vi "RT Driver VI.vi"(6 "Device Clock":string, 9 "Device Inputs FIFO":refnum<k33>, 10 "Device Outputs FIFO":refnum<k33>, 11 "Device Reference":T1 format="%.0x") -> ()   [LabVIEW 2021, in "G5 Regatron Custom Device Engine.lvlib"]
uses:
  G5 Regatron Custom Device Engine.lvlib
  <vilib>/NI VeriStand/Custom Device API/Custom Device Item Ref.ctl
  <vilib>/NI VeriStand/Custom Device API/Custom Device Channel Type.ctl
  <vilib>/Platform/TimedLoop/XDataNode/nitl_modes.ctl
  Shared/Regatron.G5.Rest Handle.llb/G5.Rest Status.ctl
  Shared/Regatron.G5.Rest System.llb/G5.Rest System Output References Datasource.ctl
  Shared/Regatron.G5.Rest System.llb/G5.Rest System Output Limits Datasource.ctl
  Shared/Regatron.G5.Rest Config.llb/G5.Rest Config Sensing Observation Datasource.ctl
  Shared/G5.Rest Battery Control Functions.ctl
  Shared/Regatron.G5.Rest System.llb/G5.Rest System Output Limits.ctl
  Shared/Regatron.G5.Rest System.llb/G5.Rest System Output References.ctl
  Shared/Regatron.G5.Rest System.llb/G5.Rest System Clear Inicidents.ctl
  Shared/Regatron.G5.Rest Config.llb/G5.Rest Sensing Observation References.ctl
  Shared/G5.Rest Battery Control Values.ctl
  <userlib>/_OpenG.lib/array/array.llb/Search 1D Array (Boolean)__ogtk.vi
  <vilib>/NI VeriStand/Custom Device API/Custom Device API.lvlib
  <vilib>/NI VeriStand/Custom Device Tools/Custom Device Utility Library/Custom Device Utility Library.lvlib
  <vilib>/Platform/TimedLoop/XDataNode/XDNodeRunTimeDep.lvlib
  Shared/Regatron.G5.Rest.lvlib
panel:
  in  "Initialization Status Notifier":refnum<notifier>
  in  "Status Notifier":refnum<notifier>
  # "Custom Device Template\nv1.0"
  # "Use this template as a starting point for creating a custom device code module. The input controls shown here are specially named controls that the system will use to provide the device loop with data. The controls are not required for the device loop to run. For instance, if the device doesn't produce any output data, then you don't need the Device Outputs FIFO control. If you do use these controls, however, they need to have these exact names to be functional."
  # "The optional status notifier element is used to notify the RT engine of the last state of the custom device, and to indicate the device has completed execution. If this control is not used, a default No Error value is returned to the system when the device finishes execution.\n\nNote: This error state is not checked until the system shuts down. Use an output status channel to send more immediate status values to the system."
  # "This optional input can be used to send the VeriStand Engine the final status of the custom device initalization process. If this control exists on the custom device front panel, the VeriStand Engine will wait for a status update before starting up. If the custom device reports an error, that will abort the execution of the current configuration in the VeriStand Engine.\n\nThis control can be deleted if the custom device does not need to send the initialization status update."
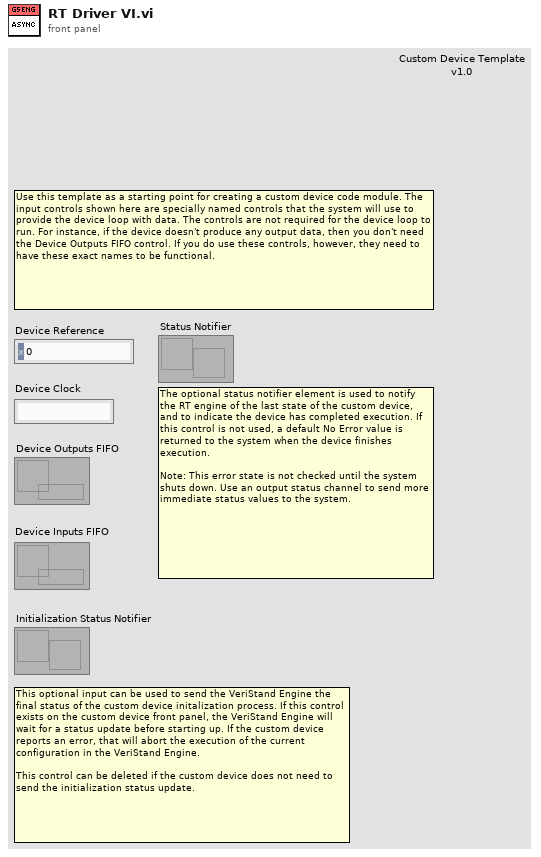
[diagram p1: front panel]
types:
  T1 = typedef "Custom Device API.lvlib/Custom Device Item Ref.ctl" = u64
  T2 = typedef "Custom Device API.lvlib/Custom Device Channel Type.ctl" = enum16{"Input", "Output"}
  T3 = typedef "Custom Device API.lvlib/Custom Device Timed Loop Priority.ctl" = enum32{"Low", "Medium", "High"}
  T4 = typedef "Regatron.G5.Rest.lvlib/G5.Rest Status.ctl" = enum16{"Read", "Write"}
  T5 = typedef "Regatron.G5.Rest.lvlib/G5.Rest Battery Control Functions.ctl" = enum16{"Read Energy Count", "Read Charge Count", "Reset Energy Charge Counters"}
  T6 = typedef "Regatron.G5.Rest.lvlib/G5.Rest System Output Limits.ctl" = cluster{"Voltage Upper Limit V":sgl, "Voltage Lower Limit V":sgl, "Current Upper Limit A":sgl, "Current Lower Limit A":sgl, "Power Upper Limit W":sgl, "Power Lower Limit W":sgl}
  T7 = typedef "Regatron.G5.Rest.lvlib/G5.Rest System Output References.ctl" = cluster{"Voltage V":sgl, "Current A":sgl, "Power W":sgl, "Load R Ohm":sgl}
  T8 = typedef "Regatron.G5.Rest.lvlib/G5.Rest System Clear Inicidents.ctl" = enum16{"Clear Errors and Warnings", "Clear Warnings", "Clear Errors"}
  T9 = typedef "Regatron.G5.Rest.lvlib/G5.Rest Sensing Observation References.ctl" = cluster{"Voltage Max Level (V)":sgl, "Voltage Max Delay (ms)":sgl}
  T10 = typedef "Regatron.G5.Rest.lvlib/G5.Rest Battery Control Values.ctl" = cluster{"Charge Counter":dbl, "Energy Counter":dbl, "ResetEnergyChargeCounters":dbl}
  T11 = typedef "XDNodeRunTimeDep.lvlib/nitl_modes.ctl" = enum32{"No Change", "Process missed periods, maintain original phase", "Discard missed periods, maintain original phase", "Process missed periods, ignore original phase", "Discard missed periods, ignore original phase"}
  T12 = typedef "Regatron.G5.Rest.lvlib/G5.Rest System Output References Datasource.ctl" = enum16{"Voltage", "Current", "Power", "Load Resistance", "ALL"}[]
  T13 = enum16{"Undefined", "PowerUp", "NotReady", "Ready", "VoltageOnPrepare", "VoltageOn", "VoltageOnLeave", "Test", "FirmwareUpdate"}
  T14 = typedef "Regatron.G5.Rest.lvlib/G5.Rest Config Quadrantmode.ctl" = enum16{"Bidirectional", "Q1 Only", "Q4 Only"}
  T15 = enum16{"VoltageControlled", "CurrentControlled", "PowerControlled", "ResistanceControlled"}
  T16 = typedef "Regatron.G5.Rest.lvlib/G5.Rest System Output Limits Datasource.ctl" = enum16{"Voltage Upper Limit", "Voltage Lower Limit", "Current Upper Limit", "Current Lower Limit", "Power Upper Limit", "Power Lower Limit", "ALL"}[]
  T17 = typedef "Regatron.G5.Rest.lvlib/G5.Rest Config Sensing Observation Datasource.ctl" = enum16{"Voltage Max Level", "Voltage Max Delay", "ALL"}[]
  T18 = typedef "Regatron.G5.Rest.lvlib/G5.Rest System Output Values.ctl" = cluster{"Voltage V":sgl, "Current A":sgl, "Power W":sgl, "Power kW":sgl, "Load R Ohm":sgl}
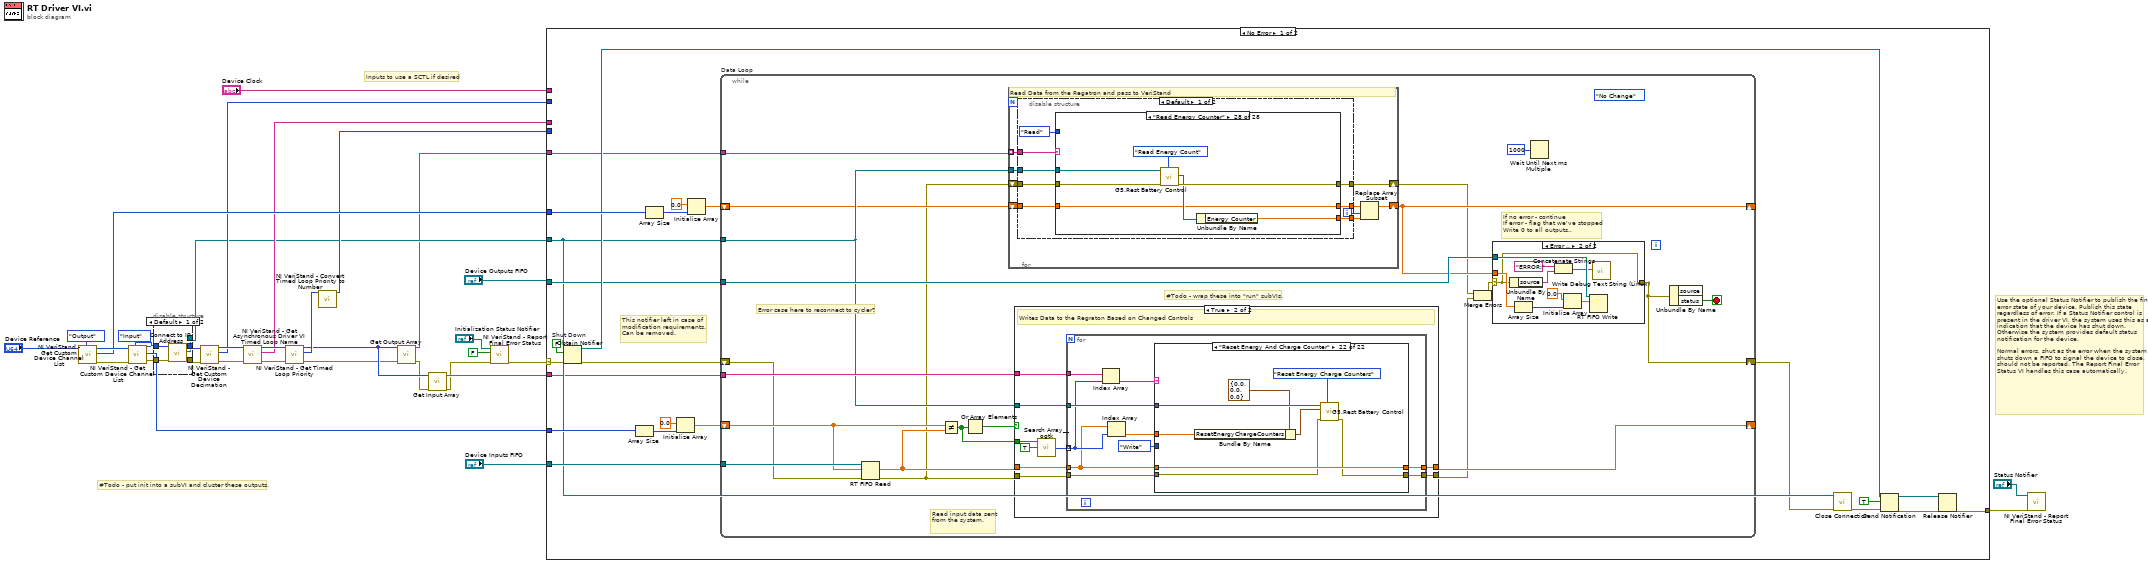
[diagram p0: block diagram]
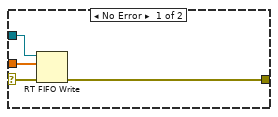
[diagram p3: hidden frame]
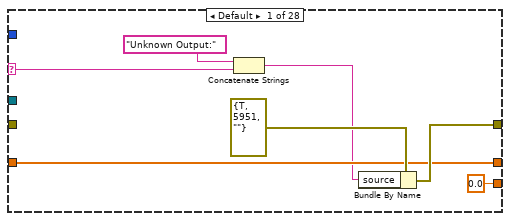
[diagram p4: hidden frame]
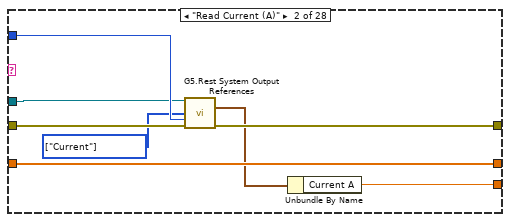
[diagram p5: hidden frame]
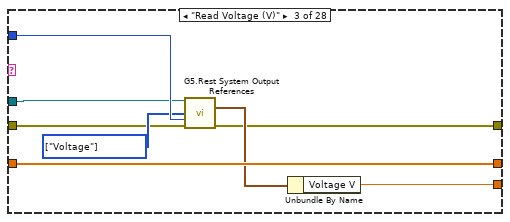
[diagram p6: hidden frame]
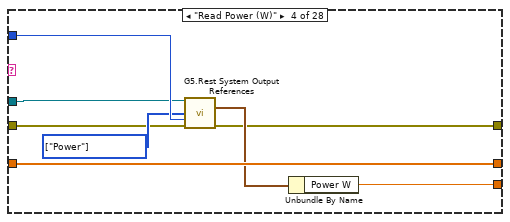
[diagram p7: hidden frame]
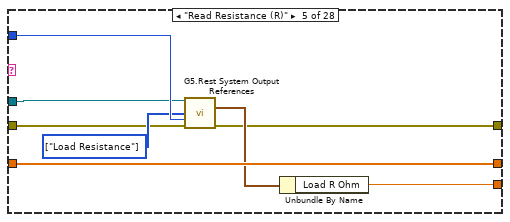
[diagram p8: hidden frame]
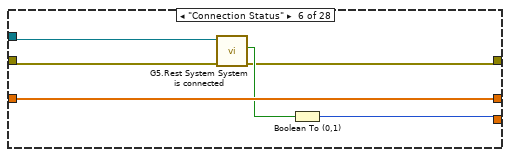
[diagram p9: hidden frame]
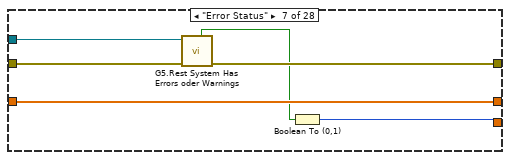
[diagram p10: hidden frame]
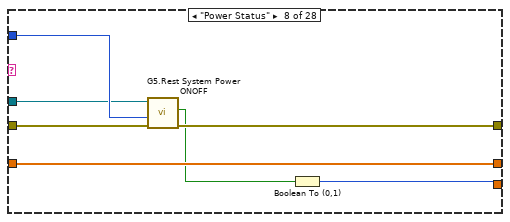
[diagram p11: hidden frame]
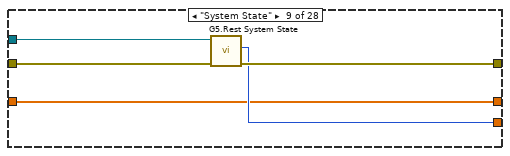
[diagram p12: hidden frame]
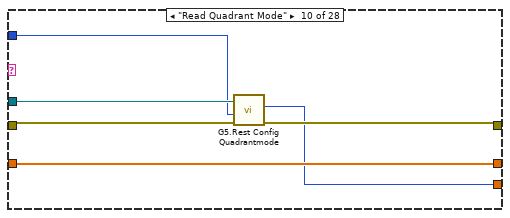
[diagram p13: hidden frame]
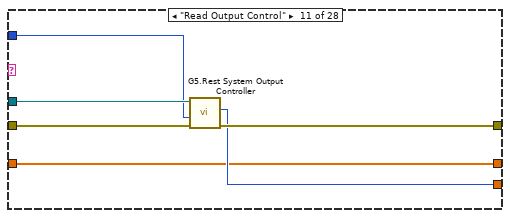
[diagram p14: hidden frame]
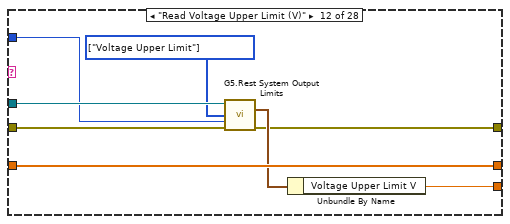
[diagram p15: hidden frame]
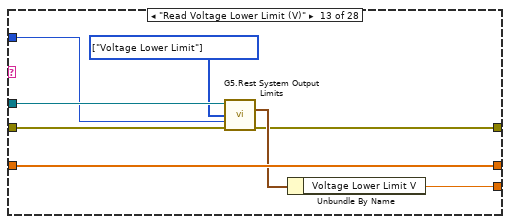
[diagram p16: hidden frame]
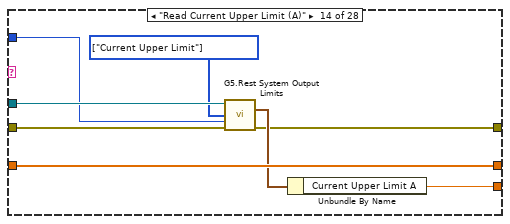
[diagram p17: hidden frame]
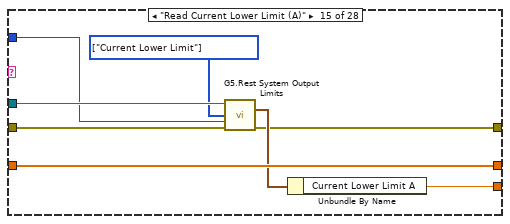
[diagram p18: hidden frame]
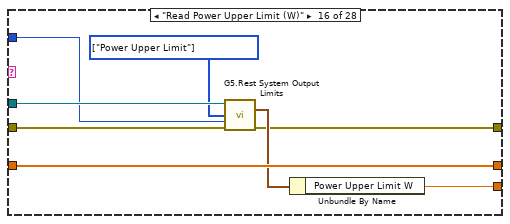
[diagram p19: hidden frame]
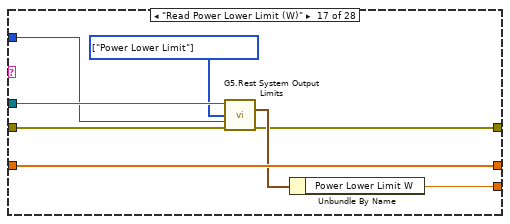
[diagram p20: hidden frame]
diagram:
  # "#Todo - put init into a subVI and cluster these outputs."
  # "Inputs to use a SCTL if desired"
  # "Use the optional Status Notifier to publish the final error state of your device. Publish this state regardless of error. If a Status Notifier control is present in the driver VI, the system uses this as an indication that the device has shut down. Otherwise the system provides default status notification for the device.\n\nNormal errors, shut as the error when the system shuts down a FIFO to signal the device to close, should not be reported. The Report Final Error Status VI handles this case automatically."
  n1 = call <vilib>:"NI VeriStand - Get Custom Device Channel List.vi"("Channel Type"=Custom_Device_Channel_Type."Output", "Device Ref in"="Device Reference") -> ("error out"=w29:errorcluster, "Specified Channel Ref List"=w26:T1[], "Device Ref out"=w30:T1)  [unwired: 1 in, 6 out]
  n2 = call <vilib>:"NI VeriStand - Get Custom Device Channel List.vi"("Channel Type"=Custom_Device_Channel_Type."Input", "error in (no error)"=w29, "Device Ref in"=w30) -> ("error out"=w22:errorcluster, "Specified Channel Ref List"=w27:T1[], "Device Ref out"=w15:T1)  [unwired: 6 out]
  n3 = disable-structure shown="Default" {
    disable-tunnel: w22 -> [w39 w40]
    disable-tunnel: [w38 w40] -> w16
    disable-tunnel: w15 -> [w37 w41]
    disable-tunnel: [w36 w41] -> w14
    disable-tunnel: [w35 _] -> w4
    frame condition #0 (active) {
      n4 = call "Connect to IP Address.vi"("error in (no error)"=w39, "Device Ref in"=w37) -> ("error out"=w38:errorcluster, "REST Client out"=w35:refnum<class "REST Client.lvclass">, "Item Ref out"=w36:T1)  [unwired: 7 in]
    }
    frame condition #1 {
    }
  }
  n5 = call <vilib>:"NI VeriStand - Get Custom Device Decimation.vi"("error in (no error)"=w16, "Device Ref in"=w14) -> ("error out"=w20:errorcluster, "Decimation"=w12:i32, "Device Ref out"=w21:T1)  [unwired: 7 in]
  n6 = call <vilib>:"NI VeriStand - Get Asynchronous Driver VI Timed Loop Name.vi"("error in (no error)"=w20, "Device Ref in"=w21) -> ("error out"=w19:errorcluster, "Device Timed Loop Name"=w11:string, "Device Ref out"=w18:T1)  [unwired: 7 in]
  n7 = call <vilib>:"NI VeriStand - Get Timed Loop Priority.vi"("error in (no error)"=w19, "Device Ref in"=w18) -> ("error out"=w8:errorcluster, "Priority"=w17:T3, "Device Ref out"=w9:T1)  [unwired: 7 in]
  n8 = call <vilib>:"NI VeriStand - Convert Timed Loop Priority to Number.vi"("Priority"=w17) -> ("Numeric Priority"=w10:i32)  [unwired: 10 in]
  n9 = call "Get Output Array.vi"("error in"=w8, "Device Ref in"=w9) -> ("error out"=w7:errorcluster, "Array"=w1:string[])  [unwired: 8 in]
  n10 = call "Get Input Array.vi"("error in"=w7, "Device Ref in"=w9) -> ("error out"=w5:errorcluster, "Array"=w6:string[])  [unwired: 8 in]
  n11 = call <vilib>:"NI VeriStand - Report Final Error Status.vi"("error in (no error)"=w5, "Filter FIFO & Shutdown Errors (T)"=FALSE ("Filter FIFO Errors (T)"), "Status Notifier"="Initialization Status Notifier") -> ("error out"=w3:errorcluster)  [unwired: 8 out]
  n12 = case shown="No Error" w3 {
    selector: w3 -> [w56 w512]
    tunnel: "Device Outputs FIFO" -> [w50 _]
    tunnel: "Device Inputs FIFO" -> [w52 _]
    tunnel: w27 -> [w61 _]
    tunnel: w26 -> [w60 _]
    tunnel: [w43 w512] -> w2
    tunnel: "Device Clock" -> [_ _]
    tunnel: w12 -> [_ _]
    tunnel: w11 -> [_ _]
    tunnel: w10 -> [_ _]
    tunnel: w1 -> [w42 _]
    tunnel: w6 -> [w44 _]
    tunnel: w4 -> [w46 _]
    frame No Error {
      w58 = FALSE  # Shut Down
      # "This notifier left in case of \nmodification requirements.\nCan be removed."
      n13 = Obtain Notifier(notification data type=w58, error in (no error)=w56) -> (notifier out=w57:refnum<notifier>, error out=w49:errorcluster)  [unwired: 2 in, 1 out]
      n14 = Array Size(array=w61) -> (size(s)=w59:i32)
      n15 = Array Size(array=w60) -> (size(s)=w62:i32)
      n16 = Initialize Array(0.0 ("element"), w59) -> (w53:dbl[])
      n17 = Initialize Array(0.0 ("element"), w62) -> (w51:dbl[])
      n18 = while "Data Loop" {
        shift-right: [w84] -> _
        shift-left: w53 -> [w81]
        shift-right: [w70] -> w45
        shift-left: w49 -> [w69]
        shift-right: [w73] -> _
        shift-left: w51 -> [w74]
        tunnel: w50 -> [w83]
        tunnel: w52 -> [w82]
        tunnel: w46 -> [w75]
        tunnel: w44 -> [w80]
        tunnel: w42 -> [w76]
        stop <- w72 stop-if-true
        (unwired) nitl_modes."No Change" ("Mode")
        # "Error case here to reconnect to cycler?"
        # "If no error - continue\nIf error - flag that we've stopped\nWrite 0 to all outputs.."
        # "#Todo - wrap these into \"run\" subVIs."
        # "Read input data sent from the system."
        n19 = RT FIFO Read(0:w82, 1:w81, 3:w69) -> (9:w78:dbl[], 11:w68:errorcluster)  [unwired: 4 out]
        n20 = Not Equal?(x=w81, y=w78) -> (x != y?=w79:bool[])
        n21 = Or Array Elements(Boolean array=w79) -> (logical OR=w77:bool)
        n22 = for {
          tunnel: w76 -> [w98] mode=indexing
          tunnel: w75 -> [w106]
          shift-right: [w105] -> w66
          shift-left: w68 -> [w103]
          shift-right: [w99] -> w73
          shift-left: w74 -> [w104]
          i -> [w101]
          # "Read Data from the Regatron and pass to VeriStand"
          n23 = disable-structure shown="Default" {
            disable-tunnel: w106 -> [w114 _]
            disable-tunnel: [w113 w315] -> w105
            disable-tunnel: w104 -> [w112 w316]
            disable-tunnel: w103 -> [w111 w315]
            disable-tunnel: [w110 w316] -> w102
            disable-tunnel: [w109 _] -> w100
            disable-tunnel: w98 -> [w107 w317]
            frame condition #0 (active) {
              n24 = case shown="\"Read Energy Counter\"" w107 {
                selector: w107 -> [w116 _ _ _ _ _ _ _ _ _ _ _ _ _ _ _ _ _ _ _ _ _ _ _ _ _ _ _]
                tunnel: w114 -> [_ w125 w131 w139 w147 w157 w163 w169 w177 w183 w189 w197 w205 w213 w221 w229 w237 w244 w249 w256 w264 w272 w279 w286 w293 w300 w307 w314]
                tunnel: w111 -> [_ w126 w132 w140 w148 w156 w162 w168 w176 w181 w188 w196 w204 w212 w220 w228 w236 w243 w248 w255 w263 w271 w278 w285 w292 w299 w305 w312]
                tunnel: [w120 w124 w130 w138 w146 w154 w161 w167 w175 w180 w186 w190 w198 w206 w214 w222 w230 w241 w247 w254 w260 w268 w277 w282 w289 w296 w304 w311] -> w113
                tunnel: w112 -> [w118 w129 w137 w145 w153 w159 w165 w172 w173 w179 w184 w193 w201 w209 w217 w225 w233 w238 w245 w251 w258 w266 w275 w280 w287 w294 w302 w309]
                tunnel: [w118 w129 w137 w145 w153 w159 w165 w172 w173 w179 w184 w193 w201 w209 w217 w225 w233 w238 w245 w251 w258 w266 w275 w280 w287 w294 w302 w309] -> w110
                tunnel: [sgl 0.0 ("Load R Ohm") w128 w135 w143 w151 w158 w164 w171 w174 w178 w185 w191 w199 w207 w215 w223 w231 w239 w246 w252 w257 w265 w276 w281 w288 w295 w301 w308] -> w109
                tunnel: G5.Rest_Status."Read" ("Status") -> [_ w127 w134 w142 w150 _ _ w170 _ w182 w187 w195 w203 w211 w219 w227 w235 w242 w250 _ w262 w270 _ _ _ _ _ _]
                frame Default {
                  n25 = Concatenate Strings("Unknown Output:" ("string"), w116) -> (w115:string)
                  n26 = Bundle By Name(cluster=errorcluster {"status"=TRUE, "code"=5951, "source"=""} ("Fehler (Ausgang)"), "source"=w115) -> (w120:errorcluster)
                }
                frame "Read Current (A)" {
                  w122 = T12 [enum."Current"] items=["Voltage", "Current", "Power", "Load Resistance", "ALL"] ("Datasource")
                  n27 = call "G5.Rest System Output References .vi"("G5 WEB API (Eingang)"=w125, "Datasource"=w122, "Status"=w127, "Fehler (Eingang, kein Fehler)"=w126) -> ("GET Output Reference"=w123:T7, "Fehler (Ausgang)"=w124:errorcluster)  [unwired: 9 in, 1 out]
                  n28 = Unbundle By Name(w123) -> ("Current A"=w128:sgl)
                }
                frame "Read Voltage (V)" {
                  w133 = T12 [enum."Voltage"] items=["Voltage", "Current", "Power", "Load Resistance", "ALL"] ("Datasource")
                  n29 = call "G5.Rest System Output References .vi"("G5 WEB API (Eingang)"=w131, "Datasource"=w133, "Status"=w134, "Fehler (Eingang, kein Fehler)"=w132) -> ("GET Output Reference"=w136:T7, "Fehler (Ausgang)"=w130:errorcluster)  [unwired: 9 in, 1 out]
                  n30 = Unbundle By Name(w136) -> ("Voltage V"=w135:sgl)
                }
                frame "Read Power (W)" {
                  w141 = T12 [enum."Power"] items=["Voltage", "Current", "Power", "Load Resistance", "ALL"] ("Datasource")
                  n31 = call "G5.Rest System Output References .vi"("G5 WEB API (Eingang)"=w139, "Datasource"=w141, "Status"=w142, "Fehler (Eingang, kein Fehler)"=w140) -> ("GET Output Reference"=w144:T7, "Fehler (Ausgang)"=w138:errorcluster)  [unwired: 9 in, 1 out]
                  n32 = Unbundle By Name(w144) -> ("Power W"=w143:sgl)
                }
                frame "Read Resistance (R)" {
                  w149 = T12 [enum."Load Resistance"] items=["Voltage", "Current", "Power", "Load Resistance", "ALL"] ("Datasource")
                  n33 = call "G5.Rest System Output References .vi"("G5 WEB API (Eingang)"=w147, "Datasource"=w149, "Status"=w150, "Fehler (Eingang, kein Fehler)"=w148) -> ("GET Output Reference"=w152:T7, "Fehler (Ausgang)"=w146:errorcluster)  [unwired: 9 in, 1 out]
                  n34 = Unbundle By Name(w152) -> ("Load R Ohm"=w151:sgl)
                }
                frame "Connection Status" {
                  n35 = call "G5.Rest System System is connected.vi"("Fehler (Eingang, kein Fehler)"=w156, "G5 WEB API (Eingang)"=w157) -> ("Fehler (Ausgang)"=w154:errorcluster, "System is connected"=w155:bool)  [unwired: 7 in, 1 out]
                  n36 = Boolean To (0,1)(Boolean=w155) -> (0, 1=w158:i16)
                }
                frame "Error Status" {
                  n37 = call "G5.Rest System Has Errors oder Warnings.vi"("Fehler (Eingang, kein Fehler)"=w162, "G5 WEB API (Eingang)"=w163) -> ("Fehler (Ausgang)"=w161:errorcluster, "System has Errors or Warnings"=w160:bool)  [unwired: 5 in, 3 out]
                  n38 = Boolean To (0,1)(Boolean=w160) -> (0, 1=w164:i16)
                }
                frame "Power Status" {
                  n39 = call "G5.Rest System Power ONOFF.vi"("Fehler (Eingang, kein Fehler)"=w168, "Status"=w170, "G5 WEB API (Eingang)"=w169) -> ("Fehler (Ausgang)"=w167:errorcluster, "Get Power OFF/ON"=w166:bool)  [unwired: 6 in, 1 out]
                  n40 = Boolean To (0,1)(Boolean=w166) -> (0, 1=w171:i16)
                }
                frame "System State" {
                  n41 = call "G5.Rest System State.vi"("Fehler (Eingang, kein Fehler)"=w176, "G5 WEB API (Eingang)"=w177) -> ("Fehler (Ausgang)"=w175:errorcluster, "GET State"=w174:T13)  [unwired: 7 in, 1 out]
                }
                frame "Read Quadrant Mode" {
                  n42 = call "G5.Rest Config Quadrantmode.vi"("Fehler (Eingang, kein Fehler)"=w181, "Status"=w182, "G5 WEB API (Eingang)"=w183) -> ("Fehler (Ausgang)"=w180:errorcluster, "GET Quadrant Mode"=w178:T14)  [unwired: 6 in, 1 out]
                }
                frame "Read Output Control" {
                  n43 = call "G5.Rest System Output Controller.vi"("Fehler (Eingang, kein Fehler)"=w188, "Status"=w187, "G5 WEB API (Eingang)"=w189) -> ("Fehler (Ausgang)"=w186:errorcluster, "GET Output Control"=w185:T15)  [unwired: 6 in, 1 out]
                }
                frame "Read Voltage Upper Limit (V)" {
                  w194 = T16 [enum."Voltage Upper Limit"] items=["Voltage Upper Limit", "Voltage Lower Limit", "Current Upper Limit", "Current Lower Limit", "Power Upper Limit", "Power Lower Limit", "ALL"] ("Datasource")
                  n44 = call "G5.Rest System Output Limits.vi"("G5 WEB API (Eingang)"=w197, "Datasource"=w194, "Status"=w195, "Fehler (Eingang, kein Fehler)"=w196) -> ("GET Output Limit"=w192:T6, "Fehler (Ausgang)"=w190:errorcluster)  [unwired: 9 in, 1 out]
                  n45 = Unbundle By Name(w192) -> ("Voltage Upper Limit V"=w191:sgl)
                }
                frame "Read Voltage Lower Limit (V)" {
                  w202 = T16 [enum."Voltage Lower Limit"] items=["Voltage Upper Limit", "Voltage Lower Limit", "Current Upper Limit", "Current Lower Limit", "Power Upper Limit", "Power Lower Limit", "ALL"] ("Datasource")
                  n46 = call "G5.Rest System Output Limits.vi"("G5 WEB API (Eingang)"=w205, "Datasource"=w202, "Status"=w203, "Fehler (Eingang, kein Fehler)"=w204) -> ("GET Output Limit"=w200:T6, "Fehler (Ausgang)"=w198:errorcluster)  [unwired: 9 in, 1 out]
                  n47 = Unbundle By Name(w200) -> ("Voltage Lower Limit V"=w199:sgl)
                }
                frame "Read Current Upper Limit (A)" {
                  w210 = T16 [enum."Current Upper Limit"] items=["Voltage Upper Limit", "Voltage Lower Limit", "Current Upper Limit", "Current Lower Limit", "Power Upper Limit", "Power Lower Limit", "ALL"] ("Datasource")
                  n48 = call "G5.Rest System Output Limits.vi"("G5 WEB API (Eingang)"=w213, "Datasource"=w210, "Status"=w211, "Fehler (Eingang, kein Fehler)"=w212) -> ("GET Output Limit"=w208:T6, "Fehler (Ausgang)"=w206:errorcluster)  [unwired: 9 in, 1 out]
                  n49 = Unbundle By Name(w208) -> ("Current Upper Limit A"=w207:sgl)
                }
                frame "Read Current Lower Limit (A)" {
                  w218 = T16 [enum."Current Lower Limit"] items=["Voltage Upper Limit", "Voltage Lower Limit", "Current Upper Limit", "Current Lower Limit", "Power Upper Limit", "Power Lower Limit", "ALL"] ("Datasource")
                  n50 = call "G5.Rest System Output Limits.vi"("G5 WEB API (Eingang)"=w221, "Datasource"=w218, "Status"=w219, "Fehler (Eingang, kein Fehler)"=w220) -> ("GET Output Limit"=w216:T6, "Fehler (Ausgang)"=w214:errorcluster)  [unwired: 9 in, 1 out]
                  n51 = Unbundle By Name(w216) -> ("Current Lower Limit A"=w215:sgl)
                }
                frame "Read Power Upper Limit (W)" {
                  w226 = T16 [enum."Power Upper Limit"] items=["Voltage Upper Limit", "Voltage Lower Limit", "Current Upper Limit", "Current Lower Limit", "Power Upper Limit", "Power Lower Limit", "ALL"] ("Datasource")
                  n52 = call "G5.Rest System Output Limits.vi"("G5 WEB API (Eingang)"=w229, "Datasource"=w226, "Status"=w227, "Fehler (Eingang, kein Fehler)"=w228) -> ("GET Output Limit"=w224:T6, "Fehler (Ausgang)"=w222:errorcluster)  [unwired: 9 in, 1 out]
                  n53 = Unbundle By Name(w224) -> ("Power Upper Limit W"=w223:sgl)
                }
                frame "Read Power Lower Limit (W)" {
                  w234 = T16 [enum."Power Lower Limit"] items=["Voltage Upper Limit", "Voltage Lower Limit", "Current Upper Limit", "Current Lower Limit", "Power Upper Limit", "Power Lower Limit", "ALL"] ("Datasource")
                  n54 = call "G5.Rest System Output Limits.vi"("G5 WEB API (Eingang)"=w237, "Datasource"=w234, "Status"=w235, "Fehler (Eingang, kein Fehler)"=w236) -> ("GET Output Limit"=w232:T6, "Fehler (Ausgang)"=w230:errorcluster)  [unwired: 9 in, 1 out]
                  n55 = Unbundle By Name(w232) -> ("Power Lower Limit W"=w231:sgl)
                }
                frame "Read Sense Enable" {
                  n56 = call "G5.Rest Config Sensing Enable.vi"("Fehler (Eingang, kein Fehler)"=w243, "Status"=w242, "G5 WEB API (Eingang)"=w244) -> ("Fehler (Ausgang)"=w241:errorcluster, "GET Voltage Sensing Enable"=w240:bool)  [unwired: 6 in, 1 out]
                  n57 = Boolean To (0,1)(Boolean=w240) -> (0, 1=w239:i16)
                }
                frame "Read Sense Max Voltage Compensation (V)" {
                  n58 = call "G5.Rest Config Sensing Compensation.vi"("Fehler (Eingang, kein Fehler)"=w248, "Status"=w250, "G5 WEB API (Eingang)"=w249) -> ("Fehler (Ausgang)"=w247:errorcluster, "GET Sense Max Voltage Compensation"=w246:sgl)  [unwired: 6 in, 1 out]
                }
                frame "Read Sense Observation Enable" {
                  n59 = call "G5.Rest Config Sensing Observing Enable.vi"("Fehler (Eingang, kein Fehler)"=w255, "G5 WEB API (Eingang)"=w256) -> ("Fehler (Ausgang)"=w254:errorcluster, "GET Sensing Observation Enable"=w253:bool)  [unwired: 7 in, 1 out]
                  n60 = Boolean To (0,1)(Boolean=w253) -> (0, 1=w252:i16)
                }
                frame "Read Sense Observation Voltage Max Level (V)" {
                  w261 = T17 [enum."Voltage Max Level"] items=["Voltage Max Level", "Voltage Max Delay", "ALL"] ("Datasource")
                  n61 = call "G5.Rest Config Sensing Observation References.vi"("G5 WEB API (Eingang)"=w264, "Datasource"=w261, "Status"=w262, "Fehler (Eingang, kein Fehler)"=w263) -> ("GET Sensing Observation References"=w259:T9, "Fehler (Ausgang)"=w260:errorcluster)  [unwired: 9 in, 1 out]
                  n62 = Unbundle By Name(w259) -> ("Voltage Max Level (V)"=w257:sgl)
                }
                frame "Read Sense Observation Voltage Max Delay (ms)" {
                  w269 = T17 [enum."Voltage Max Delay"] items=["Voltage Max Level", "Voltage Max Delay", "ALL"] ("Datasource")
                  n63 = call "G5.Rest Config Sensing Observation References.vi"("G5 WEB API (Eingang)"=w272, "Datasource"=w269, "Status"=w270, "Fehler (Eingang, kein Fehler)"=w271) -> ("GET Sensing Observation References"=w267:T9, "Fehler (Ausgang)"=w268:errorcluster)  [unwired: 9 in, 1 out]
                  n64 = Unbundle By Name(w267) -> ("Voltage Max Delay (ms)"=w265:sgl)
                }
                frame "Read Output Load R Ohm" {
                  w274 = T12 [enum."Load Resistance"] items=["Voltage", "Current", "Power", "Load Resistance", "ALL"] ("Datasource")
                  n65 = call "G5.Rest System Output Values.vi"("Fehler (Eingang, kein Fehler)"=w278, "Datasource"=w274, "G5 WEB API (Eingang)"=w279) -> ("Fehler (Ausgang)"=w277:errorcluster, "Output Values"=w273:T18)  [unwired: 6 in, 1 out]
                  n66 = Unbundle By Name(w273) -> ("Load R Ohm"=w276:sgl)
                }
                frame "Read Output Voltage (V)" {
                  w284 = T12 [enum."Voltage"] items=["Voltage", "Current", "Power", "Load Resistance", "ALL"] ("Datasource")
                  n67 = call "G5.Rest System Output Values.vi"("Fehler (Eingang, kein Fehler)"=w285, "Datasource"=w284, "G5 WEB API (Eingang)"=w286) -> ("Fehler (Ausgang)"=w282:errorcluster, "Output Values"=w283:T18)  [unwired: 6 in, 1 out]
                  n68 = Unbundle By Name(w283) -> ("Voltage V"=w281:sgl)
                }
                frame "Read Output Current (A)" {
                  w291 = T12 [enum."Current"] items=["Voltage", "Current", "Power", "Load Resistance", "ALL"] ("Datasource")
                  n69 = call "G5.Rest System Output Values.vi"("Fehler (Eingang, kein Fehler)"=w292, "Datasource"=w291, "G5 WEB API (Eingang)"=w293) -> ("Fehler (Ausgang)"=w289:errorcluster, "Output Values"=w290:T18)  [unwired: 6 in, 1 out]
                  n70 = Unbundle By Name(w290) -> ("Current A"=w288:sgl)
                }
                frame "Read Output Power (W)" {
                  w298 = T12 [enum."Power"] items=["Voltage", "Current", "Power", "Load Resistance", "ALL"] ("Datasource")
                  n71 = call "G5.Rest System Output Values.vi"("Fehler (Eingang, kein Fehler)"=w299, "Datasource"=w298, "G5 WEB API (Eingang)"=w300) -> ("Fehler (Ausgang)"=w296:errorcluster, "Output Values"=w297:T18)  [unwired: 6 in, 1 out]
                  n72 = Unbundle By Name(w297) -> ("Power W"=w295:sgl)
                }
                frame "Read Charge Counter" {
                  n73 = call "G5.Rest Battery Control.vi"("Functions"=G5.Rest_Battery_Control_Functions."Read Charge Count", "error in"=w305, "G5 WEB API in"=w307) -> ("error out"=w304:errorcluster, "BatteryControl_Data"=w303:T10)  [unwired: 6 in, 1 out]
                  n74 = Unbundle By Name(w303) -> ("Charge Counter"=w301:dbl)
                }
                frame "Read Energy Counter" {
                  n75 = call "G5.Rest Battery Control.vi"("Functions"=G5.Rest_Battery_Control_Functions."Read Energy Count", "error in"=w312, "G5 WEB API in"=w314) -> ("error out"=w311:errorcluster, "BatteryControl_Data"=w310:T10)  [unwired: 6 in, 1 out]
                  n76 = Unbundle By Name(w310) -> ("Energy Counter"=w308:dbl)
                }
              }
            }
            frame condition #1 {
              n77 = call "Write Debug Text String (Windows).vi"("text"=w317) -> ()  [unwired: 11 in]
            }
          }
          n78 = Replace Array Subset(array=w102, new element=w100, index=w101) -> (w99:dbl[])
        }
        n79 = case shown="True" w77 {
          tunnel: w75 -> [_ w328]
          tunnel: w68 -> [w319 w327]
          tunnel: w79 -> [_ w326]
          tunnel: w80 -> [_ w323]
          tunnel: [w319 w322] -> w67
          tunnel: w78 -> [w318 w321]
          tunnel: [w318 w320] -> w84
          frame False {
          }
          frame True {
            # "Writes Data to the Regraton Based on Changed Controls"
            n80 = call-poly <userlib>:"Search Array__ogtk.vi"("Array"=w326, "Element Data"=TRUE) -> ("Indices of Elements"=w324:i32[])  [unwired: 7 in]
            n81 = for {
              tunnel: w328 -> [w338]
              tunnel: w327 -> [w337]
              tunnel: w324 -> [w335] mode=indexing
              tunnel: w323 -> [w336]
              tunnel: [w333] -> w322
              tunnel: w321 -> [w332]
              tunnel: [w331] -> w320
              n82 = Index Array(array=w336, index=w335) -> (element=w329:string)
              n83 = Index Array(array=w332, index=w335) -> (element=w334:dbl)
              n84 = case shown="\"Reset Energy And Charge Counter\"" w329 {
                selector: w329 -> [w340 _ _ _ _ _ _ _ _ _ _ _ _ _ _ _ _ _ _ _ _ _]
                tunnel: w338 -> [_ w349 w353 w366 w375 w384 w393 w402 w411 w420 w429 w438 w447 w452 w460 w466 w474 w478 w487 w496 w502 w510]
                tunnel: w337 -> [_ w348 w354 w361 w370 w379 w388 w397 w406 w419 w428 w437 w446 w451 w459 w463 w473 w477 w486 w495 w501 w509]
                tunnel: w334 -> [_ w345 w356 w363 w372 w381 w390 w399 w408 w414 w423 w432 w441 _ w456 w465 w469 w481 w490 _ w499 w504]
                tunnel: [w342 w346 w352 w360 w369 w378 w387 w396 w405 w416 w425 w434 w443 w450 w454 w462 w468 w476 w485 w494 w498 w505] -> w333
                tunnel: w332 -> [w344 w350 w358 w367 w376 w385 w394 w403 w412 w421 w430 w439 w448 w453 w461 w467 w475 w484 w493 w497 w503 w511]
                tunnel: [w344 w350 w358 w367 w376 w385 w394 w403 w412 w421 w430 w439 w448 w453 w461 w467 w475 w484 w493 w497 w503 w511] -> w331
                tunnel: G5.Rest_Status."Write" ("Status") -> [_ w347 w351 w365 w374 w383 w392 w401 w410 w418 w427 w436 w445 _ w458 w464 w472 w480 w489 _ w500 _]
                frame Default {
                  w343 = errorcluster {"status"=TRUE, "code"=5952, "source"="Unknown Control Pressed"} ("Fehler (Ausgang)")
                  n85 = Unbundle By Name(w343) -> ("source"=w341:string)
                  n86 = Concatenate Strings(w340, w341) -> (w339:string)
                  n87 = Bundle By Name(cluster=w343, "source"=w339) -> (w342:errorcluster)
                }
                frame "Output Control" {
                  n88 = call "G5.Rest System Output Controller.vi"("Fehler (Eingang, kein Fehler)"=w348, "Status"=w347, "SET Output Control"=w345, "G5 WEB API (Eingang)"=w349) -> ("Fehler (Ausgang)"=w346:errorcluster)  [unwired: 5 in, 2 out]
                }
                frame "Power On/Off" {
                  n89 = Number To Boolean Array(number=w356) -> (Boolean array=w357:bool[])
                  n90 = Index Array(array=w357) -> (element=w355:bool)  [unwired: 1 in]
                  n91 = call "G5.Rest System Power ONOFF.vi"("Fehler (Eingang, kein Fehler)"=w354, "Status"=w351, "Power OFF/ON"=w355, "G5 WEB API (Eingang)"=w353) -> ("Fehler (Ausgang)"=w352:errorcluster)  [unwired: 5 in, 2 out]
                }
                frame "Current Lower Limit (A)" {
                  w359 = T16 [enum."Current Lower Limit"] items=["Voltage Upper Limit", "Voltage Lower Limit", "Current Upper Limit", "Current Lower Limit", "Power Upper Limit", "Power Lower Limit", "ALL"] ("Datasource")
                  n92 = Bundle By Name(cluster=T6 {"Voltage Upper Limit V"=0.0, "Voltage Lower Limit V"=0.0, "Current Upper Limit A"=0.0, "Current Lower Limit A"=0.0, "Power Upper Limit W"=0.0, "Power Lower Limit W"=0.0} ("SET Output Limit"), "Current Lower Limit A"=w363) -> (w362:T6)
                  n93 = call "G5.Rest System Output Limits.vi"("G5 WEB API (Eingang)"=w366, "SET Output Limit"=w362, "Datasource"=w359, "Status"=w365, "Fehler (Eingang, kein Fehler)"=w361) -> ("Fehler (Ausgang)"=w360:errorcluster)  [unwired: 8 in, 2 out]
                }
                frame "Current Upper Limit (A)" {
                  w368 = T16 [enum."Current Upper Limit"] items=["Voltage Upper Limit", "Voltage Lower Limit", "Current Upper Limit", "Current Lower Limit", "Power Upper Limit", "Power Lower Limit", "ALL"] ("Datasource")
                  n94 = Bundle By Name(cluster=T6 {"Voltage Upper Limit V"=0.0, "Voltage Lower Limit V"=0.0, "Current Upper Limit A"=0.0, "Current Lower Limit A"=0.0, "Power Upper Limit W"=0.0, "Power Lower Limit W"=0.0} ("SET Output Limit"), "Current Upper Limit A"=w372) -> (w371:T6)
                  n95 = call "G5.Rest System Output Limits.vi"("G5 WEB API (Eingang)"=w375, "SET Output Limit"=w371, "Datasource"=w368, "Status"=w374, "Fehler (Eingang, kein Fehler)"=w370) -> ("Fehler (Ausgang)"=w369:errorcluster)  [unwired: 8 in, 2 out]
                }
                frame "Power Lower Limit (W)" {
                  w377 = T16 [enum."Power Lower Limit"] items=["Voltage Upper Limit", "Voltage Lower Limit", "Current Upper Limit", "Current Lower Limit", "Power Upper Limit", "Power Lower Limit", "ALL"] ("Datasource")
                  n96 = Bundle By Name(cluster=T6 {"Voltage Upper Limit V"=0.0, "Voltage Lower Limit V"=0.0, "Current Upper Limit A"=0.0, "Current Lower Limit A"=0.0, "Power Upper Limit W"=0.0, "Power Lower Limit W"=0.0} ("SET Output Limit"), "Power Lower Limit W"=w381) -> (w380:T6)
                  n97 = call "G5.Rest System Output Limits.vi"("G5 WEB API (Eingang)"=w384, "SET Output Limit"=w380, "Datasource"=w377, "Status"=w383, "Fehler (Eingang, kein Fehler)"=w379) -> ("Fehler (Ausgang)"=w378:errorcluster)  [unwired: 8 in, 2 out]
                }
                frame "Power Upper Limit (W)" {
                  w386 = T16 [enum."Power Upper Limit"] items=["Voltage Upper Limit", "Voltage Lower Limit", "Current Upper Limit", "Current Lower Limit", "Power Upper Limit", "Power Lower Limit", "ALL"] ("Datasource")
                  n98 = Bundle By Name(cluster=T6 {"Voltage Upper Limit V"=0.0, "Voltage Lower Limit V"=0.0, "Current Upper Limit A"=0.0, "Current Lower Limit A"=0.0, "Power Upper Limit W"=0.0, "Power Lower Limit W"=0.0} ("SET Output Limit"), "Power Upper Limit W"=w390) -> (w389:T6)
                  n99 = call "G5.Rest System Output Limits.vi"("G5 WEB API (Eingang)"=w393, "SET Output Limit"=w389, "Datasource"=w386, "Status"=w392, "Fehler (Eingang, kein Fehler)"=w388) -> ("Fehler (Ausgang)"=w387:errorcluster)  [unwired: 8 in, 2 out]
                }
                frame "Voltage Lower Limit (V)" {
                  w395 = T16 [enum."Voltage Lower Limit"] items=["Voltage Upper Limit", "Voltage Lower Limit", "Current Upper Limit", "Current Lower Limit", "Power Upper Limit", "Power Lower Limit", "ALL"] ("Datasource")
                  n100 = Bundle By Name(cluster=T6 {"Voltage Upper Limit V"=0.0, "Voltage Lower Limit V"=0.0, "Current Upper Limit A"=0.0, "Current Lower Limit A"=0.0, "Power Upper Limit W"=0.0, "Power Lower Limit W"=0.0} ("SET Output Limit"), "Voltage Lower Limit V"=w399) -> (w398:T6)
                  n101 = call "G5.Rest System Output Limits.vi"("G5 WEB API (Eingang)"=w402, "SET Output Limit"=w398, "Datasource"=w395, "Status"=w401, "Fehler (Eingang, kein Fehler)"=w397) -> ("Fehler (Ausgang)"=w396:errorcluster)  [unwired: 8 in, 2 out]
                }
                frame "Voltage Upper Limit (V)" {
                  w404 = T16 [enum."Voltage Upper Limit"] items=["Voltage Upper Limit", "Voltage Lower Limit", "Current Upper Limit", "Current Lower Limit", "Power Upper Limit", "Power Lower Limit", "ALL"] ("Datasource")
                  n102 = Bundle By Name(cluster=T6 {"Voltage Upper Limit V"=0.0, "Voltage Lower Limit V"=0.0, "Current Upper Limit A"=0.0, "Current Lower Limit A"=0.0, "Power Upper Limit W"=0.0, "Power Lower Limit W"=0.0} ("SET Output Limit"), "Voltage Upper Limit V"=w408) -> (w407:T6)
                  n103 = call "G5.Rest System Output Limits.vi"("G5 WEB API (Eingang)"=w411, "SET Output Limit"=w407, "Datasource"=w404, "Status"=w410, "Fehler (Eingang, kein Fehler)"=w406) -> ("Fehler (Ausgang)"=w405:errorcluster)  [unwired: 8 in, 2 out]
                }
                frame "Current (A)" {
                  w417 = T12 [enum."Current"] items=["Voltage", "Current", "Power", "Load Resistance", "ALL"] ("Datasource")
                  n104 = Bundle By Name(cluster=T7 {"Voltage V"=0.0, "Current A"=0.0, "Power W"=0.0, "Load R Ohm"=0.0} ("SET Output Reference"), "Current A"=w414) -> (w413:T7)
                  n105 = call "G5.Rest System Output References .vi"("G5 WEB API (Eingang)"=w420, "SET Output Reference"=w413, "Datasource"=w417, "Status"=w418, "Fehler (Eingang, kein Fehler)"=w419) -> ("Fehler (Ausgang)"=w416:errorcluster)  [unwired: 8 in, 2 out]
                }
                frame "Power (W)" {
                  w426 = T12 [enum."Power"] items=["Voltage", "Current", "Power", "Load Resistance", "ALL"] ("Datasource")
                  n106 = Bundle By Name(cluster=T7 {"Voltage V"=0.0, "Current A"=0.0, "Power W"=0.0, "Load R Ohm"=0.0} ("SET Output Reference"), "Power W"=w423) -> (w422:T7)
                  n107 = call "G5.Rest System Output References .vi"("G5 WEB API (Eingang)"=w429, "SET Output Reference"=w422, "Datasource"=w426, "Status"=w427, "Fehler (Eingang, kein Fehler)"=w428) -> ("Fehler (Ausgang)"=w425:errorcluster)  [unwired: 8 in, 2 out]
                }
                frame "Resistance (R)" {
                  w435 = T12 [enum."Load Resistance"] items=["Voltage", "Current", "Power", "Load Resistance", "ALL"] ("Datasource")
                  n108 = Bundle By Name(cluster=T7 {"Voltage V"=0.0, "Current A"=0.0, "Power W"=0.0, "Load R Ohm"=0.0} ("SET Output Reference"), "Load R Ohm"=w432) -> (w431:T7)
                  n109 = call "G5.Rest System Output References .vi"("G5 WEB API (Eingang)"=w438, "SET Output Reference"=w431, "Datasource"=w435, "Status"=w436, "Fehler (Eingang, kein Fehler)"=w437) -> ("Fehler (Ausgang)"=w434:errorcluster)  [unwired: 8 in, 2 out]
                }
                frame "Voltage (V)" {
                  w444 = T12 [enum."Voltage"] items=["Voltage", "Current", "Power", "Load Resistance", "ALL"] ("Datasource")
                  n110 = Bundle By Name(cluster=T7 {"Voltage V"=0.0, "Current A"=0.0, "Power W"=0.0, "Load R Ohm"=0.0} ("SET Output Reference"), "Voltage V"=w441) -> (w440:T7)
                  n111 = call "G5.Rest System Output References .vi"("G5 WEB API (Eingang)"=w447, "SET Output Reference"=w440, "Datasource"=w444, "Status"=w445, "Fehler (Eingang, kein Fehler)"=w446) -> ("Fehler (Ausgang)"=w443:errorcluster)  [unwired: 8 in, 2 out]
                }
                frame "Clear Error" {
                  n112 = call "G5.Rest System Clear Inicidents.vi"("Fehler (Eingang, kein Fehler)"=w451, "Clear Inicidents"=G5.Rest_System_Clear_Inicidents."Clear Errors and Warnings", "G5 WEB API (Eingang)"=w452) -> ("Fehler (Ausgang)"=w450:errorcluster)  [unwired: 7 in, 1 out]
                }
                frame "Sense Enable" {
                  n113 = Number To Boolean Array(number=w456) -> (Boolean array=w457:bool[])
                  n114 = Index Array(array=w457) -> (element=w455:bool)  [unwired: 1 in]
                  n115 = call "G5.Rest Config Sensing Enable.vi"("Fehler (Eingang, kein Fehler)"=w459, "Status"=w458, "SET Voltage Sensing Enable"=w455, "G5 WEB API (Eingang)"=w460) -> ("Fehler (Ausgang)"=w454:errorcluster)  [unwired: 5 in, 2 out]
                }
                frame "Sense Max Voltage Compensation (V)" {
                  n116 = call "G5.Rest Config Sensing Compensation.vi"("Fehler (Eingang, kein Fehler)"=w463, "Status"=w464, "SET Sense Max Voltage Compensation"=w465, "G5 WEB API (Eingang)"=w466) -> ("Fehler (Ausgang)"=w462:errorcluster)  [unwired: 5 in, 2 out]
                }
                frame "Sense Observation Enable" {
                  n117 = Number To Boolean Array(number=w469) -> (Boolean array=w470:bool[])
                  n118 = Index Array(array=w470) -> (element=w471:bool)  [unwired: 1 in]
                  n119 = call "G5.Rest Config Sensing Observing Enable.vi"("Fehler (Eingang, kein Fehler)"=w473, "Status"=w472, "SET Sensing Observation Enable"=w471, "G5 WEB API (Eingang)"=w474) -> ("Fehler (Ausgang)"=w468:errorcluster)  [unwired: 5 in, 2 out]
                }
                frame "Sense Observation Voltage Max Level (V)" {
                  w479 = T17 [enum."Voltage Max Level"] items=["Voltage Max Level", "Voltage Max Delay", "ALL"] ("Datasource")
                  n120 = Bundle By Name(cluster=T9 {"Voltage Max Level (V)"=0.0, "Voltage Max Delay (ms)"=0.0} ("SET Sensing Observation References"), "Voltage Max Level (V)"=w481) -> (w482:T9)
                  n121 = call "G5.Rest Config Sensing Observation References.vi"("G5 WEB API (Eingang)"=w478, "SET Sensing Observation References"=w482, "Datasource"=w479, "Status"=w480, "Fehler (Eingang, kein Fehler)"=w477) -> ("Fehler (Ausgang)"=w476:errorcluster)  [unwired: 8 in, 2 out]
                }
                frame "Sense Observation Voltage Max Delay (ms)" {
                  w488 = T17 [enum."Voltage Max Delay"] items=["Voltage Max Level", "Voltage Max Delay", "ALL"] ("Datasource")
                  n122 = Bundle By Name(cluster=T9 {"Voltage Max Level (V)"=0.0, "Voltage Max Delay (ms)"=0.0} ("SET Sensing Observation References"), "Voltage Max Delay (ms)"=w490) -> (w491:T9)
                  n123 = call "G5.Rest Config Sensing Observation References.vi"("G5 WEB API (Eingang)"=w487, "SET Sensing Observation References"=w491, "Datasource"=w488, "Status"=w489, "Fehler (Eingang, kein Fehler)"=w486) -> ("Fehler (Ausgang)"=w485:errorcluster)  [unwired: 8 in, 2 out]
                }
                frame "Hardware Reset" {
                  n124 = call "G5.Rest System Hardware Reset.vi"("Fehler (Eingang, kein Fehler)"=w495, "G5 WEB API (Eingang)"=w496) -> ("Fehler (Ausgang)"=w494:errorcluster)  [unwired: 8 in, 1 out]
                }
                frame "Configure Quadrant Mode" {
                  n125 = call "G5.Rest Config Quadrantmode.vi"("Fehler (Eingang, kein Fehler)"=w501, "Status"=w500, "SET Quadrant Mode"=w499, "G5 WEB API (Eingang)"=w502) -> ("Fehler (Ausgang)"=w498:errorcluster)  [unwired: 5 in, 2 out]
                }
                frame "Reset Energy And Charge Counter" {
                  n126 = Bundle By Name(cluster=T10 {"Charge Counter"=0.0, "Energy Counter"=0.0, "ResetEnergyChargeCounters"=0.0} ("BatteryControl_Data"), "ResetEnergyChargeCounters"=w504) -> (w506:T10)
                  n127 = call "G5.Rest Battery Control.vi"("Functions"=G5.Rest_Battery_Control_Functions."Reset Energy Charge Counters", "error in"=w509, "BatteryControl_Data out"=w506, "G5 WEB API in"=w510) -> ("error out"=w505:errorcluster)  [unwired: 5 in, 2 out]
                }
              }
            }
          }
        }
        n128 = Merge Errors(w66, w67) -> (w65:errorcluster)
        n129 = case shown="Error .." w65 {
          selector: w65 -> [w85 w92]
          tunnel: w83 -> [w88 w94]
          tunnel: w73 -> [w87 w96]
          tunnel: [w86 w92] -> w70
          frame No Error {
            n130 = RT FIFO Write(0:w88, 1:w87, 3:w85) -> (11:w86:errorcluster)  [unwired: 1 in, 4 out]
          }
          frame Error {
            n131 = Unbundle By Name(w92) -> ("source"=w91:string)
            n132 = Array Size(array=w96) -> (size(s)=w95:i32)
            n133 = Concatenate Strings("ERROR:" ("string"), w91) -> (w90:string)
            n134 = Initialize Array(0.0, w95) -> (w93:dbl[])
            n135 = RT FIFO Write(0:w94, 1:w93) -> ()  [unwired: 2 in, 5 out]
            n136 = call "Write Debug Text String (Linux).vi"("text"=w90) -> ()  [unwired: 11 in]
          }
        }
        n137 = Wait Until Next ms Multiple(millisecond multiple=u32 1000) -> ()  [unwired: 1 out]
        n138 = Unbundle By Name(w70) -> ("status"=w72:bool)  [unwired: 1 out]
      }
      n139 = call "Close Connection.vi"("error in (no error)"=w45, "REST Client in"=w46) -> ("error out"=w47:errorcluster)  [unwired: 9 in]
      n140 = Send Notification(notification=TRUE, notifier=w57, error in (no error)=w47) -> (notifier out=w55:refnum<notifier>, error out=w48:errorcluster)
      n141 = Release Notifier(notifier=w55, error in (no error)=w48) -> (error out=w43:errorcluster)  [unwired: 1 in, 2 out]
    }
    frame Error {
    }
  }
  n142 = call <vilib>:"NI VeriStand - Report Final Error Status.vi"("error in (no error)"=w2, "Status Notifier"="Status Notifier") -> ()  [unwired: 1 in, 9 out]
